vi "ForLoopDOBlink.vi"() -> ()   [LabVIEW 2020]
uses:
  <instrlib>/HandsOnPi2040/Public/DigOuts.ctl
  <instrlib>/HandsOnPi2040/HandsOnPi2040.lvlib
panel:
  out "error out":errorcluster
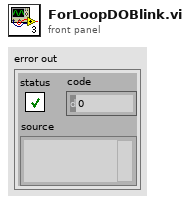
[diagram p1: front panel]
types:
  T1 = typedef "HandsOnPi2040.lvlib/DigOuts.ctl" = enum16{"No DO - Error", "DO1 (GPIO2)", "DO2 (GPIO3)", "DO3 (GPIO4)", "DO4 (GPIO5)", "BEEP (GPIO6)"}
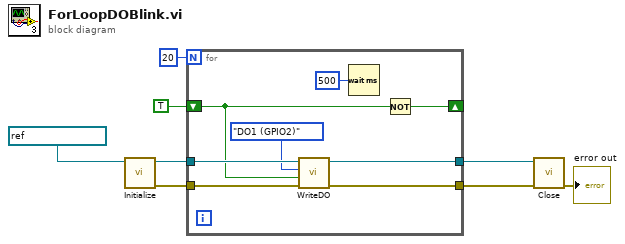
[diagram p0: block diagram]
diagram:
  n1 = call <instrlib>:"Initialize.vi"("VISA resource name"=refnum<visa-resource-name> "ASRL1::INSTR") -> ("error out"=w8:errorcluster, "VISA resource name out"=w5:refnum<visa-resource-name>)  [unwired: 8 in, 1 out]
  n2 = for {
    N: 20 -> [_]
    tunnel: w8 -> [w16]
    tunnel: [w15] -> w7
    tunnel: [w14] -> w6
    tunnel: w5 -> [w13]
    shift-right: [w12] -> _
    shift-left: TRUE -> [w11]
    n3 = call <instrlib>:"WriteDO.vi"("error in (no error)"=w16, "DO Value (True)"=w11, "Output"=DigOuts."DO1 (GPIO2)", "VISA resource name"=w13) -> ("error out"=w15:errorcluster, "VISA resource name out"=w14:refnum<visa-resource-name>)  [unwired: 6 in]
    n4 = Wait (ms)(milliseconds to wait=u32 500) -> ()  [unwired: 1 out]
    n5 = Not(x=w11) -> (.not. x?=w12:bool)
  }
  n6 = call <instrlib>:"Close.vi"("error in (no error)"=w7, "VISA resource name"=w6) -> ("error out"=→"error out":errorcluster)  [unwired: 9 in]
